vi "Get Test Registration Keys.vi"(8 "error in (no error)":errorcluster, 11 "Test Event Storage in":refnum<class "Test Event Storage.lvclass">) -> (0 "error out":errorcluster, 2 "Keys (Test IDs)":string[](array[string]), 3 "Test Event Storage out":refnum<class "Test Event Storage.lvclass">)   [LabVIEW 2013, in "Caraya.lvlib" / "Test Event Storage.lvclass"]
uses:
  Test Event Storage.lvclass
  Test Event Storage.lvclass/Test Event Storage.ctl
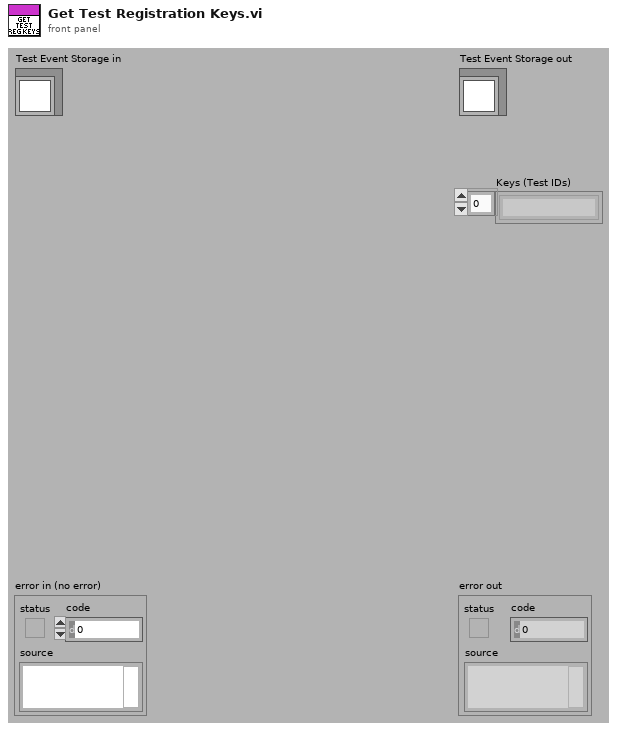
[diagram p1: front panel]
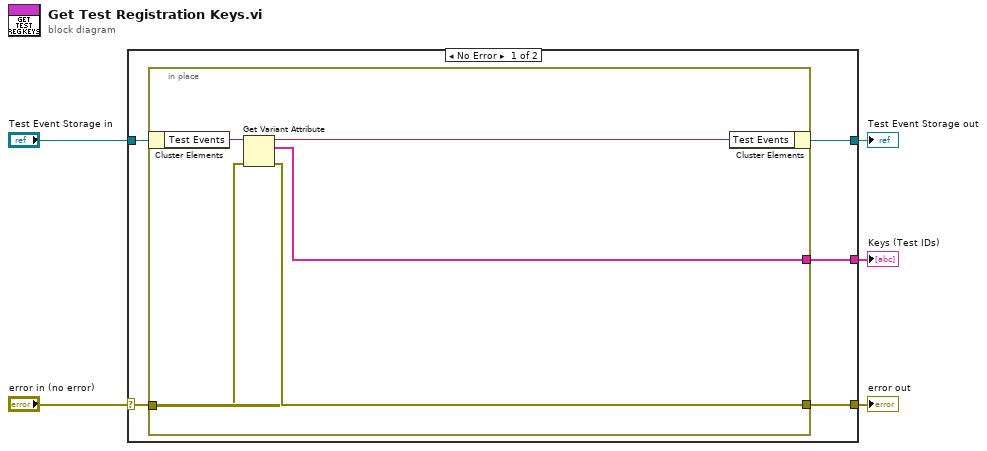
[diagram p0: block diagram]
diagram:
  n1 = case shown="No Error" "error in (no error)" {
    selector: "error in (no error)" -> [w7 w17]
    tunnel: [w10 w17] -> w4
    tunnel: [w9 w16] -> w2
    tunnel: "Test Event Storage in" -> [w8 w16]
    tunnel: [w6 _] -> w1
    frame No Error {
      n2 = in-place {
        in-place-border: w7 -> [w14]
        in-place-border: [w12] -> w10
        in-place-border: [w11] -> w6
        n3 = in-place-cluster #1(w8) -> ("Test Events"=w15:variant)
        n4 = Get Variant Attribute(Variant=w15, error in=w14) -> (duplicate Variant=w13:variant, names=w11:string[], error out=w12:errorcluster)  [unwired: 2 in, 1 out]
        n5 = in-place-cluster #1("Test Events"=w13) -> (w9:refnum<class "Test Event Storage.lvclass">)
      }
    }
    frame Error {
    }
  }
  "error out" <- w4
  "Test Event Storage out" <- w2
  "Keys (Test IDs)" <- w1
